vi "AllThingsBaxter_ROS.vi"   [LabVIEW 2013]
uses:
  BaxterVIs/Command_Joint_Angles_cluster.vi
  BaxterVIs/Read_Joint_States_A.vi
  ROS/Code/_ROSDefinition.vi
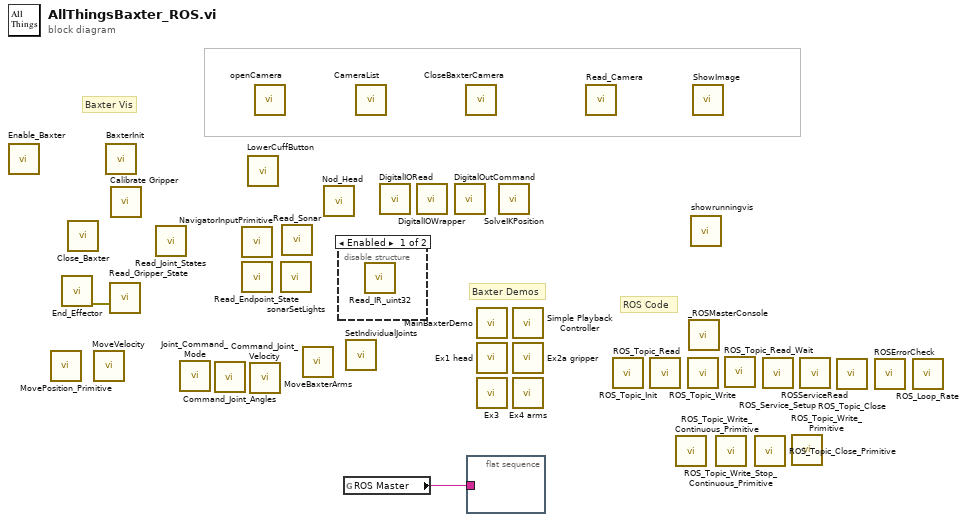
[diagram p0: block diagram]
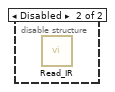
[diagram p2: hidden frame]
diagram:
  # "ROS Code"
  # "Baxter Demos"
  # "Baxter Vis"
  n1 = call "Enable_Baxter.vi"() -> ()  [unwired: 4 in, 1 out]
  n2 = call "MovePosition_Primitive.vi"() -> ()  [unwired: 6 in, 1 out]
  n3 = call "End_Effector.vi"() -> ("error out"=w1:errorcluster)  [unwired: 8 in]
  n4 = call "Close_Baxter.vi"() -> ()  [unwired: 4 in, 1 out]
  n5 = call "MoveVelocity.vi"() -> ()  [unwired: 7 in, 1 out]
  n6 = call "BaxterInit.vi"() -> ()  [unwired: 12 in]
  n7 = call "Read_Gripper_State.vi"("error in"=w1) -> ()  [unwired: 2 in, 2 out]
  n8 = call "Calibrate Gripper.vi"() -> ()  [unwired: 6 in, 1 out]
  n9 = call-poly "Read_Joint_States.vi"() -> ()  [unwired: 5 in, 4 out]
  n10 = call "Joint_Command_Mode.vi"() -> ()  [unwired: 6 in, 1 out]
  n11 = call-poly "Command_Joint_Angles.vi"() -> ()  [unwired: 9 in, 1 out]
  n12 = call "NavigatorInputPrimitive.vi"() -> ()  [unwired: 3 in, 2 out]
  n13 = call "Read_Endpoint_State.vi"() -> ()  [unwired: 3 in, 2 out]
  n14 = call "LowerCuffButton.vi"() -> ()  [unwired: 3 in, 2 out]
  n15 = call "Command_Joint_Velocity.vi"() -> ()  [unwired: 6 in, 1 out]
  n16 = call "openCamera.vi"() -> ()  [unwired: 3 in, 2 out]
  n17 = call "sonarSetLights.vi"() -> ()  [unwired: 4 in, 1 out]
  n18 = call "Read_Sonar.vi"() -> ()  [unwired: 3 in, 2 out]
  n19 = call "MoveBaxterArms.vi"() -> ()  [unwired: 6 in, 1 out]
  n20 = call "Nod_Head.vi"() -> ()  [unwired: 4 in, 1 out]
  n21 = disable-structure shown="Enabled" {
    frame Enabled {
      n22 = call "Read_IR_uint32.vi"() -> ()  [unwired: 5 in, 4 out]
    }
    frame Disabled {
      n23 = call "Read_IR.vi"() -> ()  [unwired: 3 in, 2 out]
    }
  }
  n24 = global read "_ROSDefinition.vi" "ROS Master"() -> (w2:string)
  n25 = call "SetIndividualJoints.vi"() -> ()  [unwired: 6 in, 1 out]
  n26 = call "CameraList.vi"() -> ()  [unwired: 2 in, 2 out]
  n27 = call "DigitalIORead.vi"() -> ()  [unwired: 4 in, 2 out]
  n28 = call "DigitalIOWrapper.vi"() -> ()  [unwired: 3 in, 2 out]
  n29 = call "DigitalOutCommand.vi"() -> ()  [unwired: 5 in, 1 out]
  n30 = call "CloseBaxterCamera.vi"() -> ()  [unwired: 3 in, 3 out]
  n31 = flat-sequence {
    tunnel: w2 -> [_]
    frame #0 {
    }
  }
  n32 = call "MainBaxterDemo.vi"() -> ()  [unwired: 12 in]
  n33 = call "Ex1 head.vi"() -> ()  [unwired: 12 in]
  n34 = call "Ex3.vi"() -> ()  [unwired: 12 in]
  n35 = call "SolveIKPosition.vi"() -> ()  [unwired: 7 in, 1 out]
  n36 = call "Simple Playback Controller.vi"() -> ()  [unwired: 12 in]
  n37 = call "Ex2a gripper.vi"() -> ()  [unwired: 12 in]
  n38 = call "Ex4 arms.vi"() -> ()  [unwired: 12 in]
  n39 = call "Read_Camera.vi"() -> ()  [unwired: 5 in, 3 out]
  n40 = call "ROS_Topic_Init.vi"() -> ()  [unwired: 3 in, 1 out]
  n41 = call "ROS_Topic_Read.vi"() -> ()  [unwired: 2 in, 2 out]
  n42 = call "ROS_Topic_Write_Continuous_Primitive.vi"() -> ()  [unwired: 3 in, 1 out]
  n43 = call "ROS_Topic_Write.vi"() -> ()  [unwired: 4 in, 1 out]
  n44 = call "_ROSMasterConsole.vi"() -> ()  [unwired: 12 in]
  n45 = call "showrunningvis.vi"() -> ()  [unwired: 1 in]
  n46 = call "ShowImage.vi"() -> ()  [unwired: 11 in, 1 out]
  n47 = call "ROS_Topic_Write_Stop_Continuous_Primitive.vi"() -> ()  [unwired: 3 in, 1 out]
  n48 = call "ROS_Topic_Read_Wait.vi"() -> ()  [unwired: 2 in, 2 out]
  n49 = call "ROS_Topic_Close_Primitive.vi"() -> ()  [unwired: 3 in, 1 out]
  n50 = call "ROS_Service_Setup.vi"() -> ()  [unwired: 3 in, 3 out]
  n51 = call "ROS_Topic_Write_Primitive.vi"() -> ()  [unwired: 3 in, 1 out]
  n52 = call "ROSServiceRead.vi"() -> ()  [unwired: 2 in, 3 out]
  n53 = call "ROS_Topic_Close.vi"() -> ()  [unwired: 4 in, 1 out]
  n54 = call "ROSErrorCheck.vi"() -> ()  [unwired: 3 in, 1 out]
  n55 = call "ROS_Loop_Rate.vi"() -> ()  [unwired: 5 in, 2 out]
